vi "Set_Max_Base_Values.vi"(7 "Panel In":refnum<class "Panel.lvclass">, 8 "error in (no error)":errorcluster, 9 "Basic Size New Value":dbl, 10 "Data in":T2 {"Shaft"."dmin" format="%#_7g"; "Shaft"."dmax" format="%#_7g"; "Shaft"."Fundamental Dev" format="%#_7g"; "Shaft"."Tolerance Grade (IT) Shaft" format="%#_7g"; "Hole"."Dmin" format="%#_7g"; "Hole"."Tolerance Grade (IT)" format="%#_7g"}, 11 "Base Size reference in":refnum<vi>) -> (0 "error out":errorcluster, 2 "State":T1, 3 "Data out":T2 {"Shaft"."dmin" format="%#_7g"; "Shaft"."dmax" format="%#_7g"; "Shaft"."Fundamental Dev" format="%#_7g"; "Shaft"."Tolerance Grade (IT) Shaft" format="%#_7g"; "Hole"."Dmin" format="%#_7g"; "Hole"."Tolerance Grade (IT)" format="%#_7g"})   [LabVIEW 2023]
uses:
  TypeDef/Data_Cluster.ctl
  TypeDef/Units.ctl
  TypeDef/Method_Info.ctl
  TypeDef/Hole_Data.ctl
  TypeDef/Shaft_Data.ctl
  TypeDef/State.ctl
  <vilib>/MGI/Panel Manager/Panel/Panel/Panel.lvclass
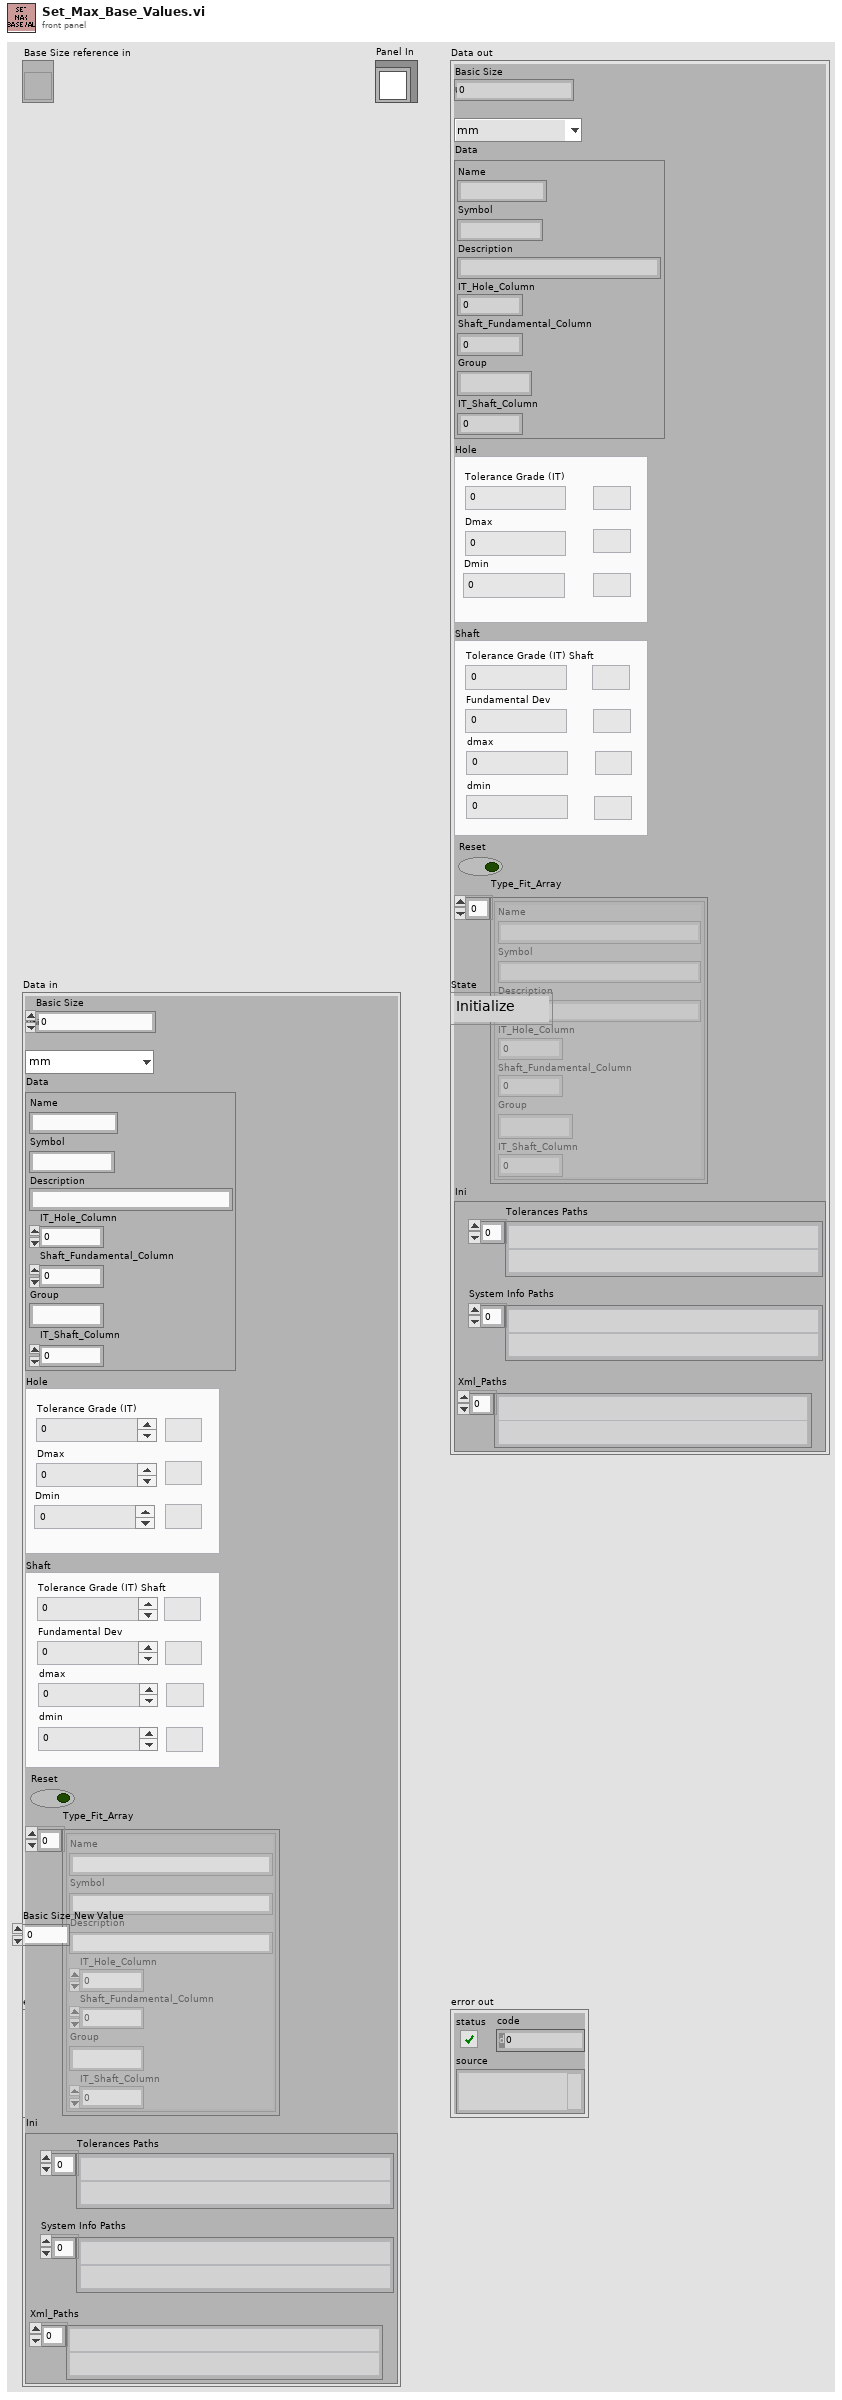
[diagram p1: front panel]
types:
  T1 = typedef "State.ctl" = enum16{"Initialize", "Wait for something", "Method_Description", "Tolerance Grade Hole", "Dmax-min", "Shaft Fudamental", "Shaft Tolerance Grade", "dmax-dmin", "Display Values"}
  T2 = typedef "Data_Cluster.ctl" = cluster{"Basic Size ":dbl, "Unit":T3, "Data":T4, "Hole":T5, "Shaft":T6, "Reset":bool, "Type_Fit_Array":T4[], "Ini":cluster{"Tolerances Paths":path[], "System Info Paths":path[], "Xml_Paths":path[]}}
  T3 = typedef "Units.ctl" = enum16{"mm", "in"}
  T4 = typedef "Method_Info.ctl" = cluster{"Name":string, "Symbol":string, "Description":string, "IT_Hole_Column":i32, "Shaft_Fundamental_Column":i32, "Group":string, "IT_Shaft_Column":i32}
  T5 = typedef "Hole_Data.ctl" = cluster{"Tolerance Grade (IT)":dbl, "Dmax":dbl, "Units Hole":cluster{"units_it":string, "units_Dmax\nUnits_Dmax":string, "Units_Dmin":string}, "Dmin":dbl}
  T6 = typedef "Shaft_Data.ctl" = cluster{"Tolerance Grade (IT) Shaft":dbl, "Units Shaft":cluster{"Units_FundamentalDev":string, "Units_dmax":string, "Units_dmin":string, "Units_IT_Shaft":string}, "Fundamental Dev":dbl, "dmax":dbl, "dmin":dbl}
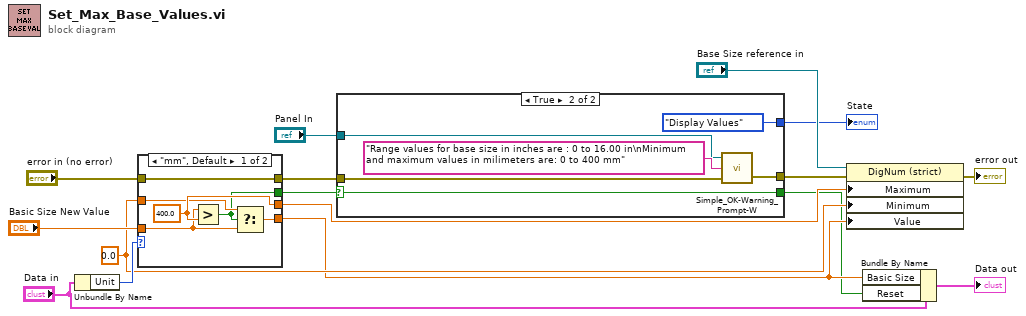
[diagram p0: block diagram]
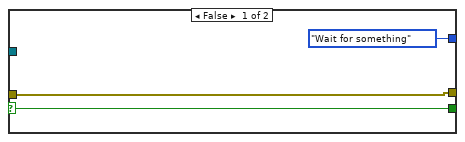
[diagram p2: hidden frame]
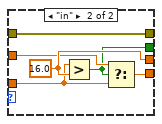
[diagram p3: hidden frame]
diagram:
  w8 = 0.0 ("Data Entry Limits:Minimum")
  n1 = Unbundle By Name("Data in") -> ("Unit"=w14:T3)
  n2 = case shown="\"mm\", Default" w14 {
    tunnel: [w20 w27] -> w16
    tunnel: "error in (no error)" -> [w22 w28]
    tunnel: [w22 w28] -> w6
    tunnel: "Basic Size New Value" -> [w18 w24]
    tunnel: [w21 w26] -> w4
    tunnel: w8 -> [w19 w25]
    tunnel: [w17 w23] -> w7
    frame "mm", Default {
      w20 = 400.0 ("Data Entry Limits:Maximum")
      n3 = Greater?(x=w18, y=w20) -> (0:w17:bool)
      n4 = Select(t=w19, s=w17, f=w18) -> (s? t:f=w21:dbl)
    }
    frame "in" {
      w27 = 16.0 ("Data Entry Limits:Maximum")
      n5 = Greater?(x=w24, y=w27) -> (0:w23:bool)
      n6 = Select(t=w25, s=w23, f=w24) -> (s? t:f=w26:dbl)
    }
  }
  n7 = case shown="True" w7 {
    selector: w7 -> [w30 w37]
    tunnel: w6 -> [w31 w35]
    tunnel: [w31 w34] -> w5
    tunnel: [w30 w37] -> w3
    tunnel: [State."Wait for something" State."Display Values"] -> w2
    tunnel: "Panel In" -> [_ w32]
    frame False {
    }
    frame True {
      n8 = call "Simple_OK-Warning_Prompt-W.vi"("error in"=w35, "User Message In"="Range values for base size in inches are : 0 to 16.00 in\nMinimum and maximum values in milimeters are: 0 to 400 mm", "Panel In"=w32) -> ("error out"=w34:errorcluster)  [unwired: 2 in]
    }
  }
  "State" <- w2
  n9 = property on="Property Node" class="DigNum (strict)"(reference="Base Size reference in", error in=w5, "Maximum"=w16, "Minimum"=w8, "Value"=w4) -> (error out=→"error out":errorcluster)  [unwired: 1 out]
  n10 = Bundle By Name(cluster="Data in", "Basic Size"=w4, "Reset"=w3) -> (→"Data out":T2)
